vi "Read Data.vi"(8 "error in (no error)":errorcluster, 11 "ControlDragStartingMsg In":refnum<class "ControlDragStartingMsg.lvclass">) -> (0 "error out":errorcluster, 2 "Data":T1(array[cluster]), 3 "ControlDragStartingMsg Out":refnum<class "ControlDragStartingMsg.lvclass">)   [LabVIEW 2017, in "ActorEvents.lvlib" / "ControlDragStartingMsg.lvclass"]
uses:
  ControlDragStartingMsg.lvclass
  ControlDragStartingMsg.lvclass/ControlDragStartingMsg.ctl
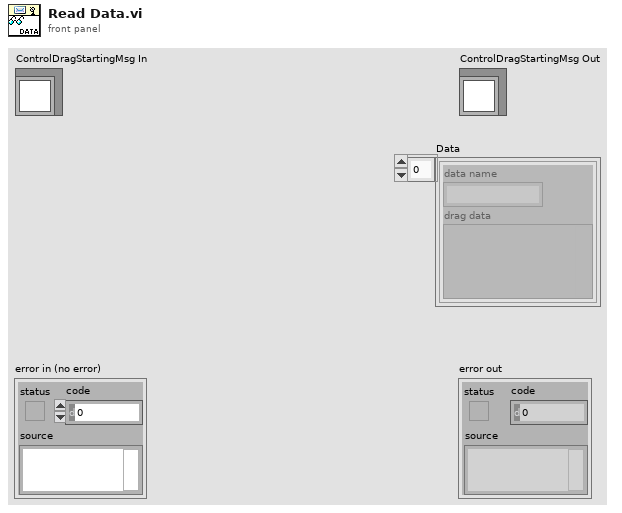
[diagram p1: front panel]
types:
  T1 = cluster{"data name":string, "drag data":variant}[]
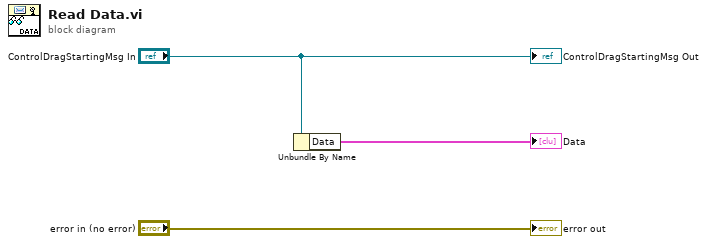
[diagram p0: block diagram]
diagram:
  n1 = Unbundle By Name("ControlDragStartingMsg In") -> ("Data"=→"Data":T1)
  "error out" <- "error in (no error)"
  "ControlDragStartingMsg Out" <- "ControlDragStartingMsg In"
